vi "m9003monitor.vi"() -> ()   [LabVIEW 2009]
panel:
  in  "Timeout (ms)":u32=60000
  in  "Channel (1 or 2)":u8=1
  out "Handle":i32
  in  "Photons per sample":u32=50
  out "Cps (current)":dbl[unit] format="%#_7g"
  in  "PMT on?":bool
  out "Cps (average)":dbl[unit] format="%#_7g"
  out "M9003":T1
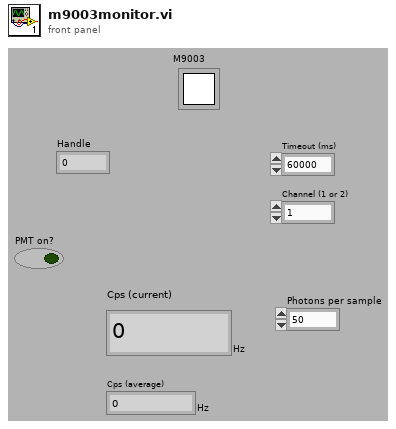
[diagram p1: front panel]
types:
  T1 = typedef "Semaphore RefNum" = refnum<k1>
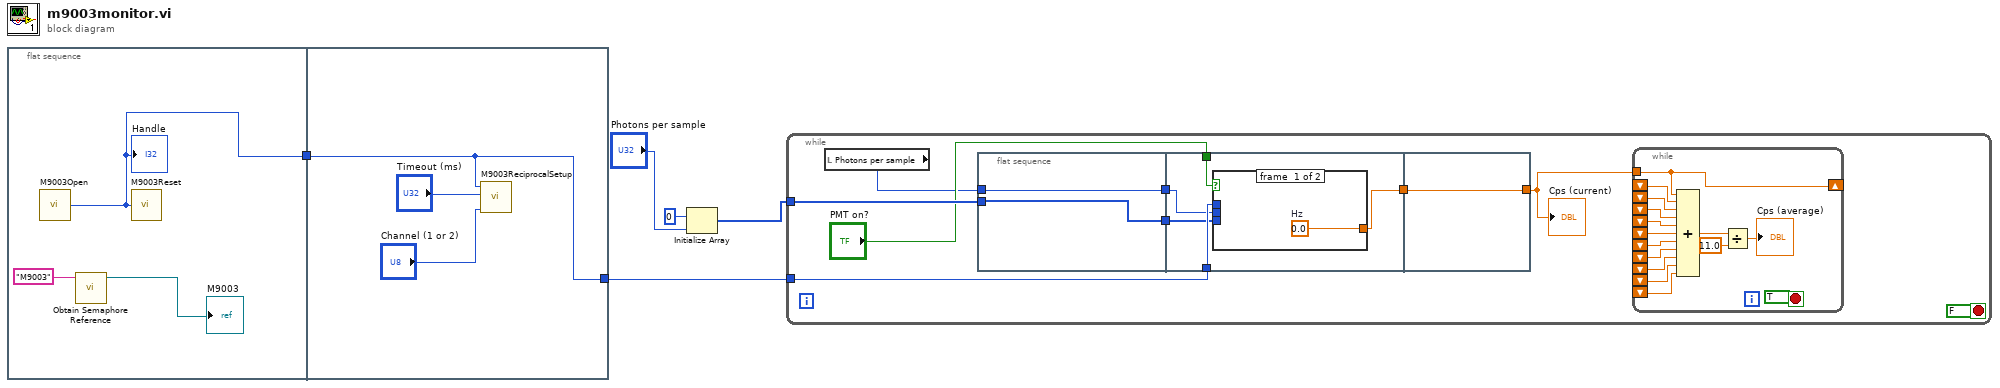
[diagram p0: block diagram]
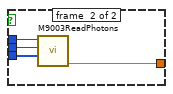
[diagram p2: hidden frame]
diagram:
  n1 = flat-sequence {
    tunnel: [w6] -> w2
    tunnel: w2 -> [w9]
    tunnel: [w9] -> w1
    frame #0 {
      n2 = call "M9003Open.vi"() -> ("HANDLE"=w6:i32)
      "Handle" <- w6
      n3 = call <vilib>:"Obtain Semaphore Reference.vi"("name (unnamed)"="M9003") -> ("semaphore"=→"M9003":T1)  [unwired: 4 in, 2 out]
      n4 = call "M9003Reset.vi"("HANDLE"=w6) -> ()
    }
    frame #1 {
      n5 = call "M9003ReciprocalSetup.vi"("Channel (default 1)"="Channel (1 or 2)", "Timeout (0=no timeout)"="Timeout (ms)", "HANDLE"=w9) -> ()  [unwired: 9 in]
    }
  }
  n6 = Initialize Array(u32 0, "Photons per sample") -> (w3:u32[])
  n7 = while {
    tunnel: w1 -> [w19]
    tunnel: w3 -> [w18]
    stop <- FALSE stop-if-true
    n8 = local read "Photons per sample"() -> (w12:u32)
    n9 = flat-sequence {
      tunnel: w12 -> [w36]
      tunnel: w18 -> [w37]
      tunnel: [w37] -> w17
      tunnel: [w36] -> w16
      tunnel: w19 -> [w42]
      tunnel: w17 -> [w41]
      tunnel: w16 -> [w40]
      tunnel: [w39] -> w15
      tunnel: "PMT on?" -> [w38]
      tunnel: [w48] -> w13
      tunnel: w15 -> [w48]
      frame #0 {
      }
      frame #1 {
        n10 = case shown="True" w38 {
          tunnel: w42 -> [_ w47]
          tunnel: w41 -> [_ w46]
          tunnel: w40 -> [_ w45]
          tunnel: [w43 w44] -> w39
          frame #0 {
            w43 = dbl[unit] 0.0  # Hz
          }
          frame #1 {
            n11 = call "M9003ReadPhotons.vi"("Prealocaed Data"=w46, "Number of Photons"=w45, "HANDLE"=w47) -> ("Photons/Second"=w44:dbl[unit])  [unwired: 5 in, 3 out]
          }
        }
      }
      frame #2 {
      }
    }
    n12 = while {
      shift-right: [w34] -> _
      shift-left: _ -> [w33]
      shift-left: _ -> [w32]
      shift-left: _ -> [w31]
      shift-left: _ -> [w30]
      shift-left: _ -> [w29]
      shift-left: _ -> [w28]
      shift-left: _ -> [w27]
      shift-left: _ -> [w26]
      shift-left: _ -> [w25]
      shift-left: _ -> [w24]
      tunnel: w13 -> [w34]
      stop <- TRUE stop-if-true
      n13 = Compound Arithmetic op=ADD(w34, w33, w32, w31, w30, w29, w28, w27, w26, w25, w24) -> (w23:dbl[unit])
      n14 = Divide(x=w23, y=11.0) -> (x/y=→"Cps (average)":dbl[unit])
    }
    "Cps (current)" <- w13
  }
